vi "Simulation - Tank Level Win SW demo2.vi"() -> ()   [LabVIEW 2025]
doc: "This example demonstrates a process simulation for a tank level. The process has added noise, valve deadband, lag, and deadtime. A level controller adjusts the inflow to a tank. An on/off valve serves as a drain that you can click on to operate. This s-valve represents a change in the process loading. You also can switch this VI from automatic control to manual control."
uses:
  <vilib>/addons/control/pid/pid.llb/PID Advanced (DBL).vi
  <vilib>/addons/control/pid/NI_PID_pid.lvlib
panel:
  in  "Physical Model":bool=TRUE
  in  "Tab Control":enum32{"Introduction", "Operation"}(tab)=enum."Operation"
  out "Flow sensor":bool
  in  "HV-101":bool
  out "tank level":dbl(slide) scale=0.0..100.0 scale format="%#.2g"
  out "Valve":bool
  in  "LCV-101":dbl(knob) scale=0.0..100.0
  in  "Auto":bool=TRUE
  out "Process Chart":T1(graph)={"initial PV"=18.934717983735947, "SP(%)"=34.59119496855346, "output"=100.0}
  in  "Setpoint":dbl(slide)=50.0 scale=0.0..100.0
  in  "PID parameters (LIC 101)":T2={"Kc"=10.0, "Ti (min)"=0.05, "Td (min)"=0.0} {"Td (min)" format="%#.6f"; "Ti (min)" format="%#.4f"; "Kc" format="%#.4f"}
  in  "Stop":bool
  # "Tank Level Control"
  # "Overview: This example demonstrates a process simulation for a tank level.  The process has added noise, valve deadband, lag, and deadtime.  A level controller adjusts the inflow to a tank.  An on/off valve serves as a drain that you can click on to operate.  This s-valve represents a change in the process loading.  You also can switch this VI from automatic control to manual control.\nInstructions:\n1. Run the VI.\n2. Verify the PID controller in closed-loop to track the setpoint.\n3. Change the setpoint to another value and verify the controller tracking the new setpoint.\n4. Apply a disturbance to the system by switching the valve HV 102 (click on the valve symbol). You will see the controller recovering fro the change.\n5. Change PID gains and see if you can improve its performance without going unstable.\n6. Switch to manual mode and see if you can control the level by changing the Valve LVC 101.\n7. Click Stop to stop the VI."
  # "ISA Symbology: The diagram uses the ISA Symbology used for control"
  # "Loop 101"
  # "Level Controller at the control room"
  # "Level Transmitter on the field"
  # "Level Control Valve on the field"
  # "Hand Control Valve on the field"
  # "HV"
  # "102"
  # "LCV"
  # "101"
  # "LIC"
  # "101"
  # "LT"
  # "101"
  # "Slow Leak"
  # "Click to operate"
  # "HV"
  # "102"
  # "LCV"
  # "101"
  # "LIC"
  # "101"
  # "LT"
  # "101"
  # "Manual"
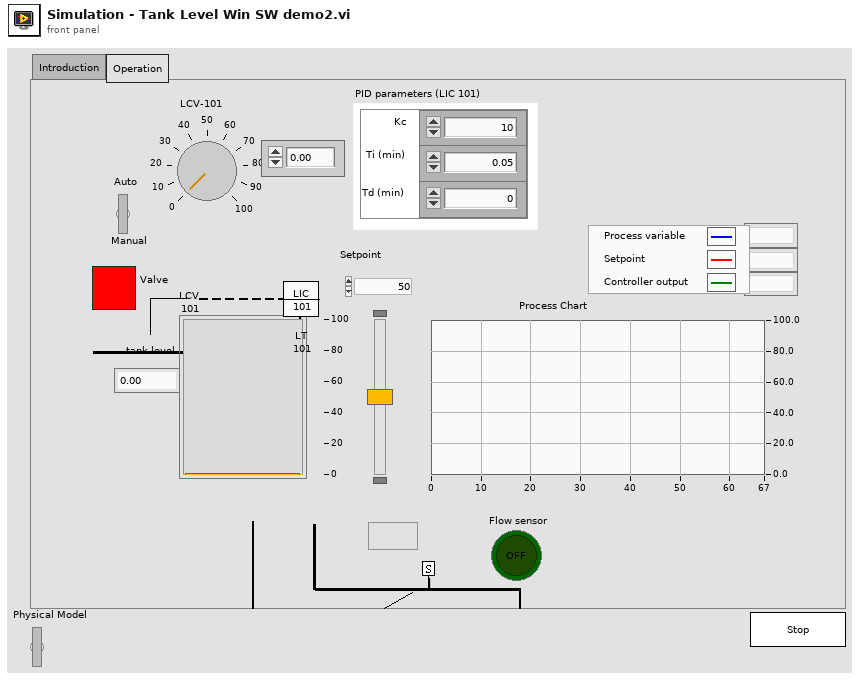
[diagram p1: front panel]
types:
  T1 = cluster{"initial PV":dbl, "SP(%)":dbl, "output":dbl}
  T2 = cluster{"Kc":dbl, "Ti (min)":dbl, "Td (min)":dbl}
  T3 = cluster{"static gain":dbl, "lag (s)":dbl, "deadtime (s)":dbl, "load":dbl, "deadband":dbl, "sensor noise":dbl, "initial PV":dbl, "plant noise":dbl}
  T4 = cluster{"Plant Output":dbl, "Setpoint":dbl, "output":dbl}
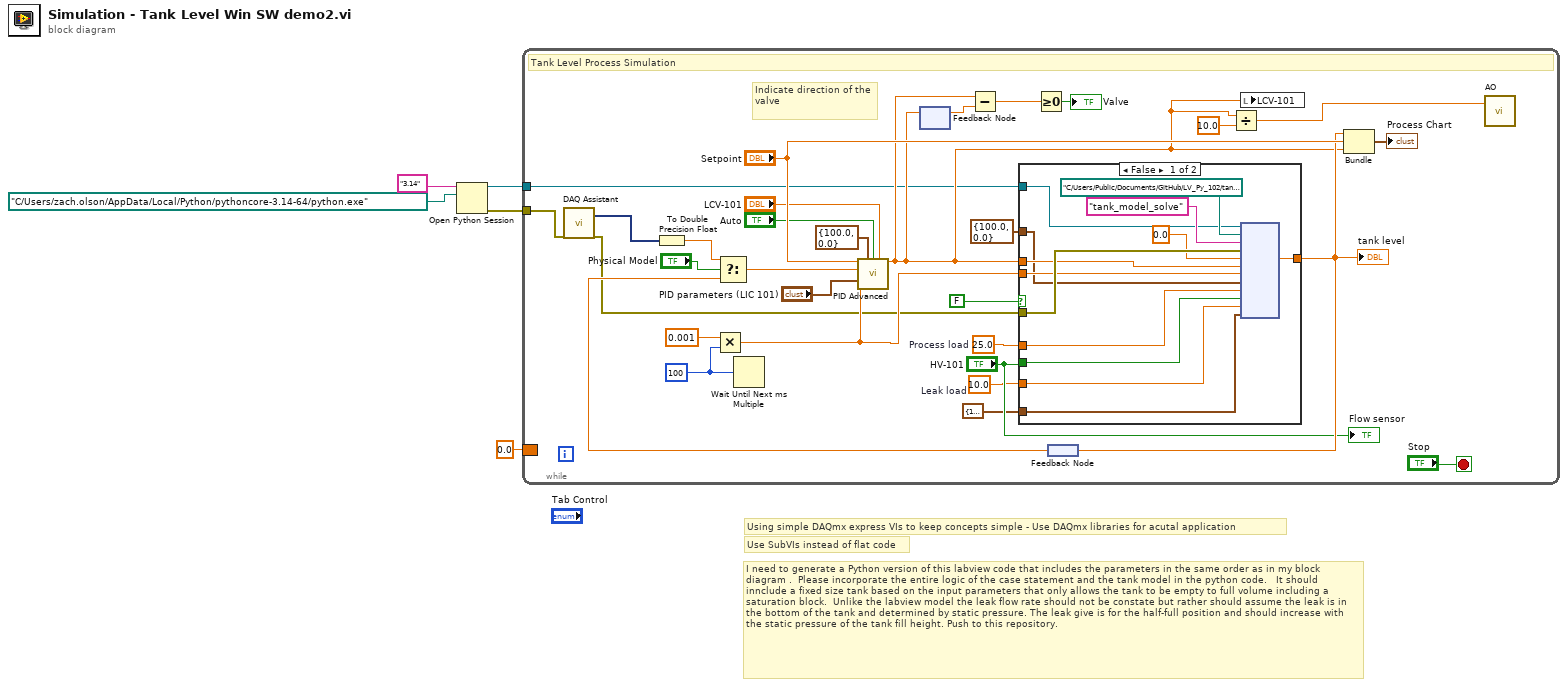
[diagram p0: block diagram]
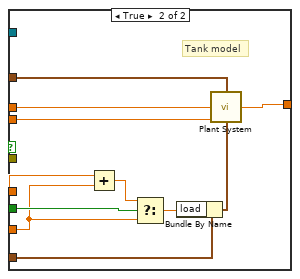
[diagram p2: hidden frame]
diagram:
  # "I need to generate a Python version of this labview code that includes the parameters in the same order as in my block diagram .  Please incorporate the entire logic of the case statement and the tank model in the python code.   It should innclude a fixed size tank based on the input parameters that only allows the tank to be empty to full volume including a saturation block.  Unlike the labview model the leak flow rate should not be constate but rather should assume the leak is in the bottom of the tank and determined by static pressure. The leak give is for the half-full position and should increase with the static pressure of the tank fill height. Push to this repository."
  # "Use SubVIs instead of flat code"
  # "Using simple DAQmx express VIs to keep concepts simple - Use DAQmx libraries for acutal application"
  n1 = Open Python Session(python version="3.14" ("Python version"), python path=path "C:/Users/zach.olson/AppData/Local/Python/pythoncore-3.14-64/python.exe" ("Python path")) -> (session out=w2:refnum<k35>, error out=w1:errorcluster)  [unwired: 1 in]
  n2 = while {
    border: 0.0 ("Plant Output") -> [_]
    tunnel: w2 -> [w13]
    tunnel: w1 -> [w12]
    stop <- "Stop" stop-if-true
    w8 = 25.0  # Process load
    w9 = 10.0  # Leak load
    w28 = u32 100
    # "Indicate direction of the valve"
    # "Tank Level Process Simulation"
    n3 = call "DAQ Assistant"("error in"=w12) -> ("data"=w14:dynamicdata, "error out"=w11:errorcluster)  [unwired: 16 in, 1 out]
    n4 = To Double Precision Float(number=w14) -> (double precision float=w15:dbl)
    n5 = Multiply(x=0.001, y=w28) -> (x*y=w27:dbl)
    n6 = Wait Until Next ms Multiple(millisecond multiple=w28) -> ()  [unwired: 1 out]
    n7 = feedback #1() -> (w25:dbl)  [unwired: 1 in]
    n8 = feedback #2() -> (w17:dbl)
    n9 = Select(t=w15, s="Physical Model", f=w17) -> (s? t:f=w18:dbl)
    n10 = call-poly <vilib>:"PID Advanced.vi"("setpoint"="Setpoint", "output range"=cluster{"output high":dbl, "output low":dbl} {"output high"=100.0, "output low"=0.0}, "auto? (T)"="Auto", "manual control"="LCV-101", "process variable"=w18, "PID gains"="PID parameters (LIC 101)", "dt (s)"=w27) -> ("output"=w21:dbl)  [unwired: 7 in, 1 out]
    n11 = feedback-in #1(w21) -> ()
    n12 = Subtract(x=w21, y=w25) -> (x-y=w24:dbl)
    n13 = case shown="False" FALSE {
      tunnel: w27 -> [w44 w58]
      tunnel: [w37 w57] -> w26
      tunnel: "HV-101" -> [w40 w55]
      tunnel: w21 -> [w45 w54]
      tunnel: w13 -> [w47 _]
      tunnel: w11 -> [w46 _]
      tunnel: w9 -> [w39 w53]
      tunnel: w8 -> [w41 w52]
      tunnel: cluster{"output high":dbl, "output low":dbl} {"output high"=100.0, "output low"=0.0} ("output saturation range") -> [w42 w51]
      tunnel: T3 {"static gain"=1.5, "lag (s)"=18.0, "deadtime (s)"=1.0, "load"=0.0, "deadband"=1.0, "sensor noise"=0.0, "initial PV"=0.0, "plant noise"=5.0} ("process parameters") -> [w38 w50]
      frame False {
        n14 = node(w47, path "C:/Users/Public/Documents/GitHub/LV_Py_102/tank.py" ("module path"), "tank_model_solve" ("function name"), w46, 0.0 ("output low"), w45, w44, w42, w41, w40, w39, w38) -> (w37:dbl)  [unwired: 7 in, 4 out]
      }
      frame True {
        # "Tank model"
        n15 = Add(x=w52, y=w53) -> (x+y=w56:dbl)
        n16 = Select(t=w56, s=w55, f=w53) -> (s? t:f=w60:dbl)
        n17 = Bundle By Name(cluster=w50, "load"=w60) -> (w59:T3)
        n18 = call "Plant System.vi"("output saturation range"=w51, "Plant Input"=w54, "dt (s)"=w58, "process parameters"=w59) -> ("Plant Output"=w57:dbl)  [unwired: 11 in]
      }
    }
    "tank level" <- w26
    n19 = Greater Or Equal To 0?(x=w24) -> (x >= 0?=→"Valve":bool)
    n20 = feedback-in #2(w26) -> ()
    n21 = Divide(x=w21, y=10.0) -> (x/y=w19:dbl)
    n22 = local write "LCV-101"(w21) -> ()
    n23 = Bundle("Plant Output"=w26, "Setpoint"="Setpoint", "output"=w21) -> (→"Process Chart":T4)  [unwired: 1 in]
    n24 = call "AO"("data"=w19) -> ()  [unwired: 17 in, 2 out]
    "Flow sensor" <- "HV-101"
  }
